vi "Disable All Digital Modulation.vi"(8 "error in (no error)":errorcluster, 11 "VISA resource name":refnum<visa-resource-name>) -> (0 "error out":errorcluster, 3 "VISA resource name out":refnum<visa-resource-name>)   [LabVIEW 2011, in "Agilent PSG MXG Series.lvlib"]
doc: "Disables all digital modulation personalities on a particular baseband. It does not affect analog modulation.\n\n<B>Notes:</B>\n(1) This VI is valid only in E8267C, E8267D, N5182A.\n\n(2) For E8267C, this VI is valid only when the instrument installs <B>Option 002</B> (Internal baseband generator) or <B>Option 602</B> (Digital bus baseband generator).\n\n(3) For E8267D, this VI is valid only when the instrument installs <B>Option 601</B> or <B>Option 602</B> (Internal baseband generator).\n\n(4) For E5182A, this VI is valid only when the instrument installs <B>Option 651</B> or <B>Option 652</B> or <B>Option 654</B> (Internal baseband generator)."
uses:
  Agilent PSG MXG Series.lvlib
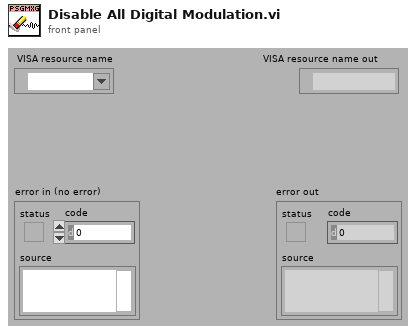
[diagram p1: front panel]
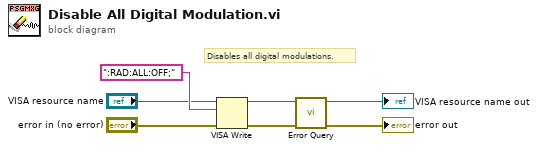
[diagram p0: block diagram]
diagram:
  # "Disables all digital modulations."
  n1 = VISA Write(VISA resource name="VISA resource name", write buffer=":RAD:ALL:OFF;", error in (no error)="error in (no error)") -> (VISA resource name out=w6:refnum<visa-resource-name>, error out=w5:errorcluster)  [unwired: 1 out]
  n2 = call "Error Query.vi"("error in (no error)"=w5, "VISA resource name"=w6) -> ("error out"=→"error out":errorcluster, "VISA resource name out"=→"VISA resource name out":refnum<visa-resource-name>)  [unwired: 6 in, 2 out]
